vi "readFromXML.vi"(8 "error in (no error)":errorcluster, 10 "XML in":string, 11 "ProperMotion in":refnum<class "ProperMotion.lvclass">) -> (0 "error out":errorcluster, 3 "ProperMotion out":refnum<class "ProperMotion.lvclass">)   [LabVIEW 2014, in "TCSDataDefinitions.lvlib" / "TCSCommand.lvlib" / "TargetConfiguration.lvlib" / "Target.lvlib" / "FixedTarget.lvlib" / "ProperMotion.lvclass"]
uses:
  ProperMotion.lvclass
  <userlib>/Common/UnitsAndXML/FlattenItemWithUnitToXML/FlattenAngularVelocityToXML/AngularVelocityUnit.ctl
  ProperMotion.lvclass/ProperMotion.ctl
  <userlib>/Common/UnitsAndXML/UnitsAndXML.lvlib
  <userlib>/Common/XML/XMLParser/XMLParser.lvclass
panel:
  out "pmDec_masPYr":dbl[unit]
  out "pmRA_masPYr":dbl[unit]
  out "epochPM_Yr":dbl
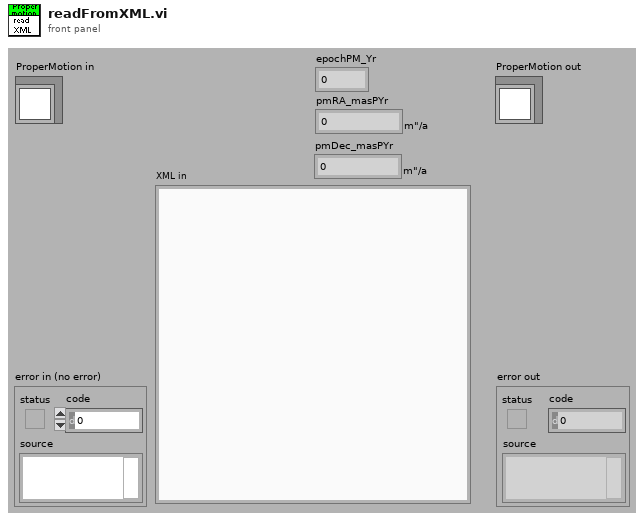
[diagram p1: front panel]
types:
  T1 = typedef "UnitsAndXML.lvlib/AngularVelocityUnit.ctl" = enum16{"\"/a", "deg/s", "\"/s"}
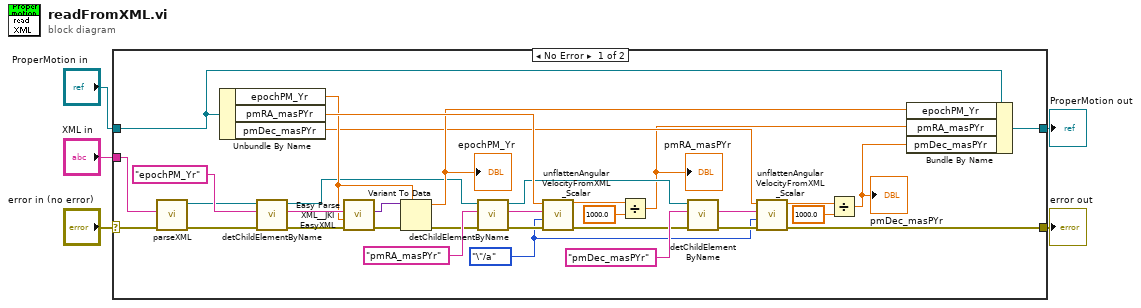
[diagram p0: block diagram]
diagram:
  n1 = case shown="No Error" "error in (no error)" {
    selector: "error in (no error)" -> [w36 w40]
    tunnel: [w15 w40] -> w4
    tunnel: [w30 w39] -> w2
    tunnel: "ProperMotion in" -> [w31 w39]
    tunnel: "XML in" -> [w38 _]
    frame No Error {
      w13 = AngularVelocityUnit."\"/a" ("angularVelocityUnitInXML")
      n2 = call <userlib>:"parseXML.vi"("error in (no error)"=w36, "XMLString in"=w38) -> ("error out"=w37:errorcluster, "Element out"=w20:refnum<class "XMLParser.lvclass">)  [unwired: 8 in]
      n3 = Unbundle By Name(w31) -> ("epochPM_Yr"=w23:dbl, "pmRA_masPYr"=w29:dbl[unit], "pmDec_masPYr"=w12:dbl[unit])
      n4 = call <userlib>:"detChildElementByName.vi"("error in (no error)"=w37, "childName"="epochPM_Yr" ("ChildName"), "Element in"=w20) -> ("error out"=w25:errorcluster, "childXML"=w24:string, "Element out"=w19:refnum<class "XMLParser.lvclass">)  [unwired: 5 in, 1 out]
      n5 = call <vilib>:"Easy Parse XML__JKI EasyXML.vi"("error in (no error)"=w25, "LabVIEW Data (Type)"=w23, "XML String"=w24) -> ("error out"=w32:errorcluster, "LabVIEW Data"=w17:variant)  [unwired: 7 in]
      n6 = Variant To Data(error in=w32, type=w23, Variant=w17) -> (data=w22:dbl, error out=w21:errorcluster)
      "epochPM_Yr" <- w22
      n7 = call <userlib>:"detChildElementByName.vi"("error in (no error)"=w21, "childName"="pmRA_masPYr" ("ChildName"), "Element in"=w19) -> ("error out"=w27:errorcluster, "childXML"=w28:string, "Element out"=w18:refnum<class "XMLParser.lvclass">)  [unwired: 5 in, 1 out]
      n8 = call <userlib>:"unflattenAngularVelocityFromXML_Scalar.vi"("error in (no error)"=w27, "angularVelocityUnitInXML"=w13, "xmlString"=w28, "angularVelocityForType"=w29) -> ("error out"=w26:errorcluster, "angularVelocity"=w10:dbl[unit])  [unwired: 6 in]
      n9 = Divide(x=w10, y=1000.0) -> (x/y=w11:dbl[unit])
      "pmRA_masPYr" <- w11
      n10 = call <userlib>:"detChildElementByName.vi"("error in (no error)"=w26, "childName"="pmDec_masPYr" ("ChildName"), "Element in"=w18) -> ("error out"=w16:errorcluster, "childXML"=w14:string)  [unwired: 5 in, 2 out]
      n11 = call <userlib>:"unflattenAngularVelocityFromXML_Scalar.vi"("error in (no error)"=w16, "angularVelocityUnitInXML"=w13, "xmlString"=w14, "angularVelocityForType"=w12) -> ("error out"=w15:errorcluster, "angularVelocity"=w8:dbl[unit])  [unwired: 6 in]
      n12 = Divide(x=w8, y=1000.0) -> (x/y=w6:dbl[unit])
      "pmDec_masPYr" <- w6
      n13 = Bundle By Name(cluster=w31, "epochPM_Yr"=w22, "pmRA_masPYr"=w11, "pmDec_masPYr"=w6) -> (w30:refnum<class "ProperMotion.lvclass">)
    }
    frame Error {
    }
  }
  "error out" <- w4
  "ProperMotion out" <- w2
